vi "PAQ_Table_read_n_samples.vi"(8 "error in (no error)":errorcluster, 9 "Sub Path":path, 10 "Required samples":i32, 11 "Table Filename":string) -> (0 "error out":errorcluster, 1 "TAGs":string[](array[string]), 2 "Fetched samples":i32, 3 "value":T1)   [LabVIEW 2020, in "Sgraph_lib_V1.lvlib" / "DBAL-BIN.lvclass"]
uses:
  DBAL-BIN.lvclass
  controls/BIN/BINdata.ctl
  Common/controls/Global-test.vi
  Builds/Sgraph_lib_V1.lvlib
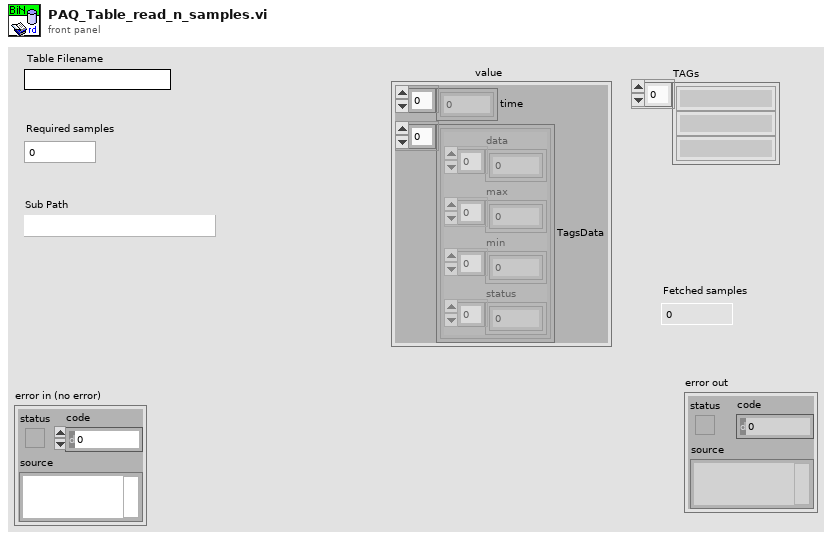
[diagram p1: front panel]
types:
  T1 = typedef "Sgraph_lib_V1.lvlib/DBAL-BIN.lvclass/BINdata.ctl" = cluster{"time":dbl[], "TagsData":cluster{"data":dbl[], "max":dbl[], "min":dbl[], "status":u32[]}[]}
  T2 = cluster{"data":dbl[], "max":dbl[], "min":dbl[], "status":u32[]}[]
  T3 = cluster{"data":dbl[], "max":dbl[], "min":dbl[], "status":u32[]}
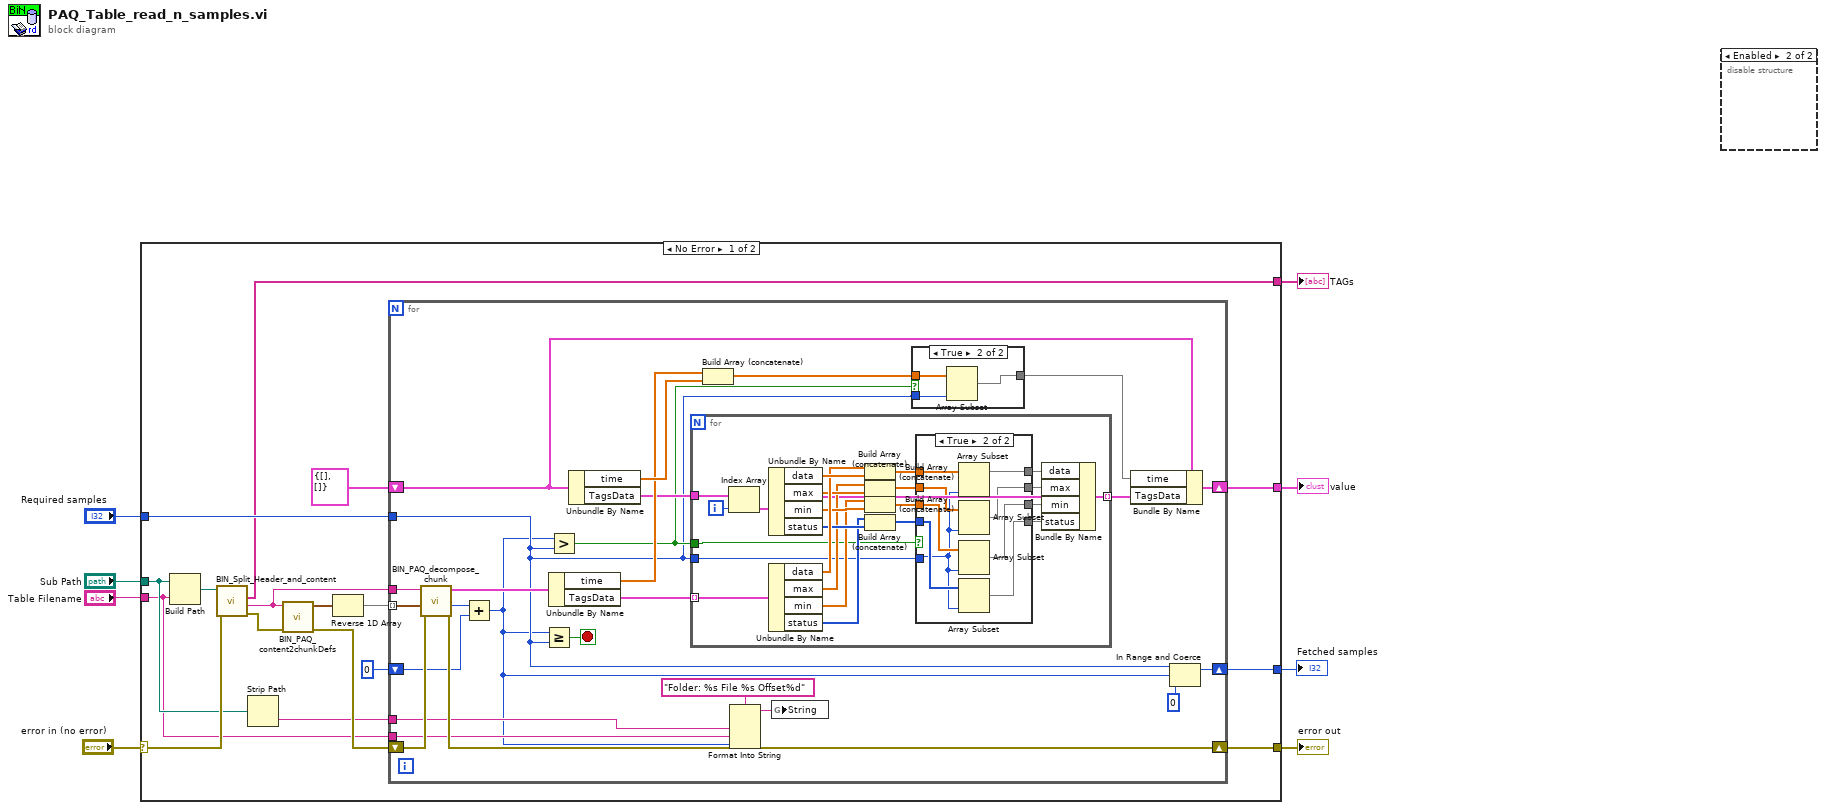
[diagram p0: block diagram]
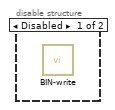
[diagram p2: hidden frame]
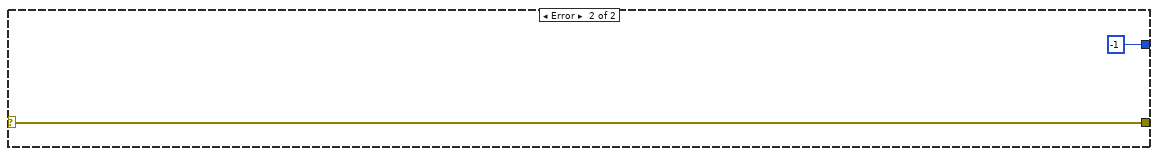
[diagram p5: hidden frame]
diagram:
  n1 = case shown="No Error" "error in (no error)" {
    selector: "error in (no error)" -> [w24 w93]
    tunnel: [w20 w93] -> w7
    tunnel: "Sub Path" -> [w11 _]
    tunnel: "Table Filename" -> [w9 _]
    tunnel: "Required samples" -> [w18 _]
    tunnel: [w14 -1 ("Samples size")] -> w1
    tunnel: [w13 _] -> w3
    tunnel: [w12 _] -> w2
    frame No Error {
      n2 = Build Path(base path=w11, name or relative path=w9) -> (appended path=w25:path)
      n3 = call "BIN_Split_Header_and_content.vi"("error in"=w24, "Path in"=w25) -> ("error out"=w23:errorcluster, "Content"=w22:string, "TAGs"=w12:string[])  [unwired: 5 in, 2 out]
      n4 = Strip Path(path=w11) -> (name=w10:string)  [unwired: 1 out]
      n5 = call "BIN_PAQ_content2chunkDefs.vi"("error in (no error)"=w23, "Content"=w22) -> ("error out"=w21:errorcluster, "Data segments"=w19:cluster{"Offset":u32, "Size":u32}[])  [unwired: 8 in]
      n6 = Reverse 1D Array(array=w19) -> (reversed array=w17:cluster{"Offset":u32, "Size":u32}[])
      n7 = for {
        tunnel: w17 -> [w51] mode=indexing
        tunnel: w22 -> [w50]
        shift-right: [w48] -> w20
        shift-left: w21 -> [w49]
        tunnel: w18 -> [w31]
        shift-right: [w35] -> w14
        shift-left: 0 ("Samples size") -> [w36]
        shift-right: [w45] -> w13
        shift-left: T1 {"time"=[], "TagsData"=[]} ("PAQ_data") -> [w47]
        tunnel: w10 -> [w28]
        tunnel: w9 -> [w27]
        stop <- w39 stop-if-true
        n8 = call "BIN_PAQ_decompose_chunk.vi"("error in (no error)"=w49, "Offset"=w51, "Content"=w50) -> ("error out"=w48:errorcluster, "Samples size"=w37:i32, "PAQ_data"=w46:T1)  [unwired: 6 in]
        n9 = Add(x=w37, y=w36) -> (x+y=w26:i32)
        n10 = Greater Or Equal?(x=w26, y=w31) -> (x >= y?=w39:bool)
        n11 = Greater?(x=w26, y=w31) -> (0:w34:bool)
        n12 = Unbundle By Name(w46) -> ("time"=w43:dbl[], "TagsData"=w42:T2)
        n13 = Unbundle By Name(w47) -> ("time"=w44:dbl[], "TagsData"=w41:T2)
        n14 = for {
          tunnel: w42 -> [w76] mode=indexing
          tunnel: w41 -> [w78]
          tunnel: [w66] -> w40 mode=indexing
          tunnel: w34 -> [w65]
          tunnel: w31 -> [w56]
          i -> [w77]
          n15 = Index Array(array=w78, index=w77) -> (element=w67:T3)
          n16 = Unbundle By Name(w67) -> ("data"=w75:dbl[], "max"=w73:dbl[], "min"=w72:dbl[], "status"=w71:u32[])
          n17 = Unbundle By Name(w76) -> ("data"=w74:dbl[], "max"=w68:dbl[], "min"=w69:dbl[], "status"=w70:u32[])
          n18 = Build Array (concatenate)(w74, w75) -> (w64:dbl[])
          n19 = Build Array (concatenate)(w68, w73) -> (w63:dbl[])
          n20 = Build Array (concatenate)(w69, w72) -> (w61:dbl[])
          n21 = Build Array (concatenate)(w70, w71) -> (w62:u32[])
          n22 = case shown="True" w65 {
            tunnel: w64 -> [w80 w91]
            tunnel: w63 -> [w81 w89]
            tunnel: w62 -> [w79 w85]
            tunnel: w61 -> [w82 w86]
            tunnel: [w82 w87] -> w60
            tunnel: [w81 w88] -> w59
            tunnel: [w80 w90] -> w58
            tunnel: [w79 w84] -> w57
            tunnel: w56 -> [_ w83]
            frame False {
            }
            frame True {
              n23 = Array Subset(array=w91, length=w83) -> (w90:dbl[])  [unwired: 1 in]
              n24 = Array Subset(array=w89, length=w83) -> (w88:dbl[])  [unwired: 1 in]
              n25 = Array Subset(array=w86, length=w83) -> (w87:dbl[])  [unwired: 1 in]
              n26 = Array Subset(array=w85, length=w83) -> (w84:u32[])  [unwired: 1 in]
            }
          }
          n27 = Bundle By Name(cluster=w67, "data"=w58, "max"=w59, "min"=w60, "status"=w57) -> (w66:T3)
        }
        n28 = Build Array (concatenate)(w43, w44) -> (w33:dbl[])
        n29 = Format Into String(format string="Folder: %s File %s Offset%d", w28, w27, w26) -> (resulting string=w30:string)  [unwired: 2 in, 1 out]
        n30 = global write "Global-test.vi" "String"(w30) -> ()
        n31 = case shown="True" w34 {
          tunnel: w33 -> [w52 w55]
          tunnel: [w52 w54] -> w32
          tunnel: w31 -> [_ w53]
          frame False {
          }
          frame True {
            n32 = Array Subset(array=w55, length=w53) -> (w54:dbl[])  [unwired: 1 in]
          }
        }
        n33 = Bundle By Name(cluster=w47, "time"=w32, "TagsData"=w40) -> (w45:T1)
        n34 = In Range and Coerce(upper limit=w31, x=w26, lower limit=0) -> (coerced(x)=w35:i32)  [unwired: 1 out]
      }
    }
    frame Error {
    }
  }
  "error out" <- w7
  "Fetched samples" <- w1
  "TAGs" <- w2
  "value" <- w3
  n35 = disable-structure shown="Enabled" {
    frame Disabled {
      n36 = call "BIN-write.vi"() -> ()  [unwired: 9 in, 3 out]
    }
    frame Enabled {
    }
  }
